vi "CfgManager.Text.INI Test Launcher.vi"() -> ()   [LabVIEW 2013]
uses:
  source/Manager.Text.INI/ConfigManager.Text.INI.lvclass
  <vilib>/LabVIEW Open Source Project/Data Manipulation/TypeDescriptor/TypeDescriptor_GetName.vi
  <vilib>/LabVIEW Open Source Project/Data Manipulation/TypeDescriptor/TypeDescriptor_GetPString.vi
  source/Manager/Decompose KVPs.vi
  source/Manager/Write.vi
  source/Manager/ConfigManager.lvclass
  <vilib>/LabVIEW Open Source Project/Data Manipulation/Variant/OpenVariant.lvlib
panel:
  out "Settings":cluster{"P":dbl, "I":dbl, "D":dbl}
  out "_staticdeps":T1
  out "any found?":bool
  out "_dyndependencies":T2(array[cluster])
  out "Keys":string[](array[string])
  out "modified configuration":variant
  out "error out":errorcluster
  out "initial configuration":variant
  out "filepath":path
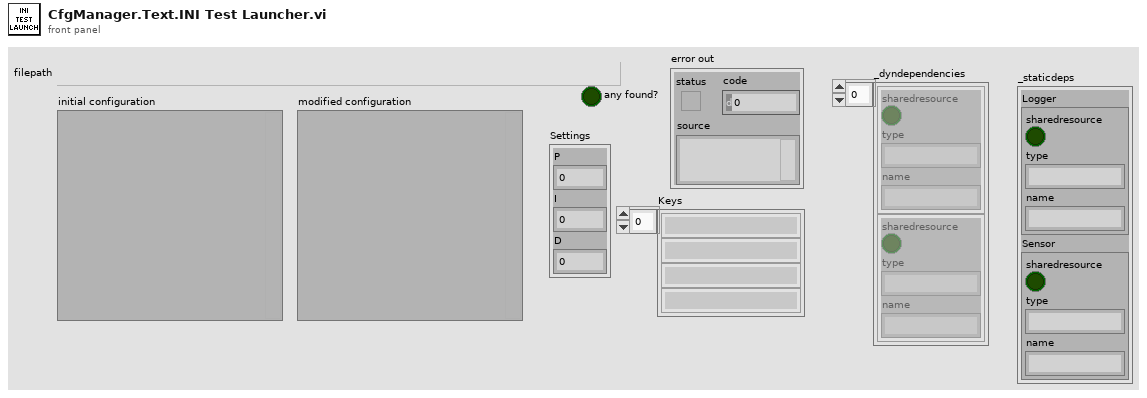
[diagram p1: front panel]
types:
  T1 = cluster{"Logger":cluster{"sharedresource":bool, "type":string, "name":string}, "Sensor":cluster{"sharedresource":bool, "type":string, "name":string}}
  T2 = cluster{"sharedresource":bool, "type":string, "name":string}[]
  T3 = cluster{"sharedresource":bool, "type":string, "name":string}
  T4 = cluster{"String":string, "Numeric":dbl, "Boolean":bool}
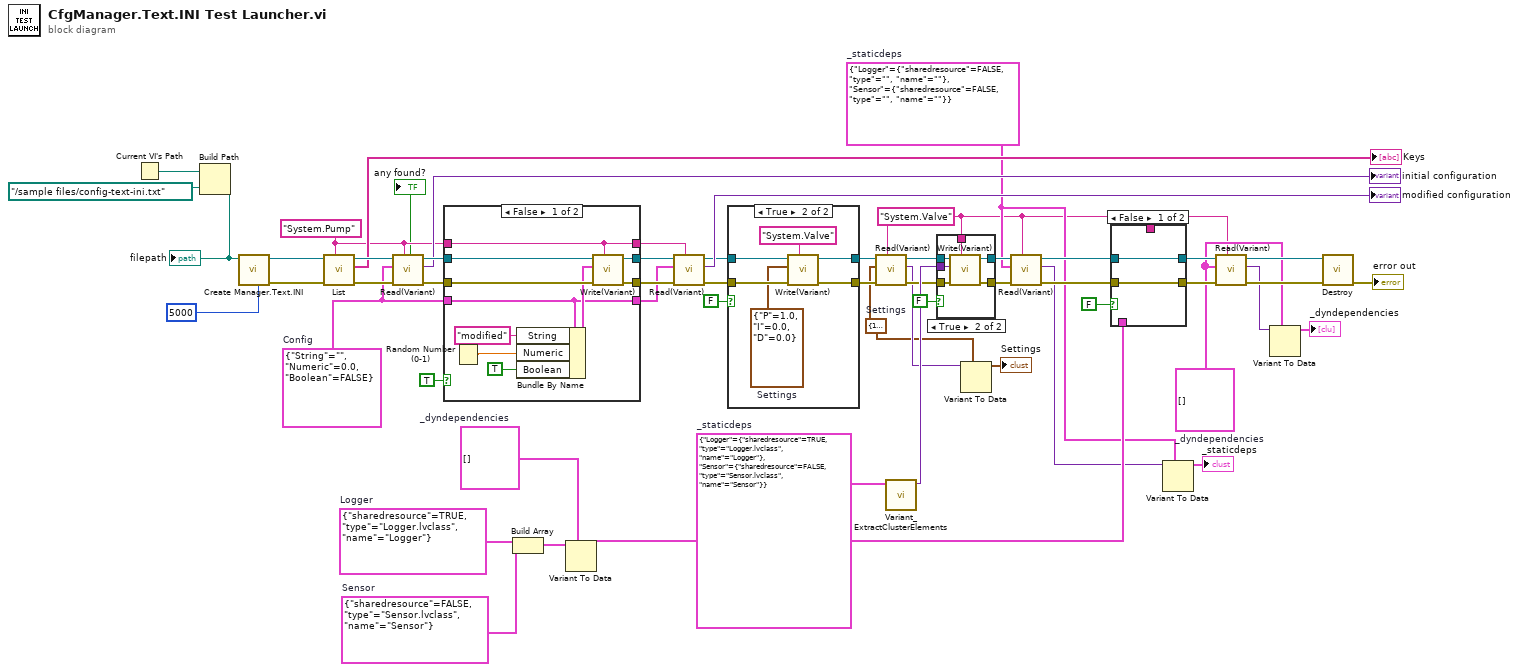
[diagram p0: block diagram]
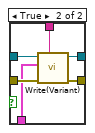
[diagram p3: hidden frame]
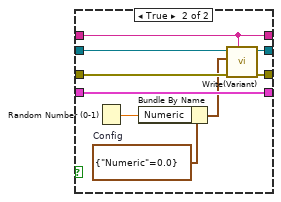
[diagram p4: hidden frame]
diagram:
  w2 = cluster{"P":dbl, "I":dbl, "D":dbl} {"P"=1.0, "I"=0.0, "D"=0.0}  # Settings
  w11 = T1 {"Logger"={"sharedresource"=FALSE, "type"="", "name"=""}, "Sensor"={"sharedresource"=FALSE, "type"="", "name"=""}}  # _staticdeps
  w21 = T2 []  # _dyndependencies
  w27 = T2 []  # _dyndependencies
  w29 = T3 {"sharedresource"=FALSE, "type"="Sensor.lvclass", "name"="Sensor"}  # Sensor
  w30 = T3 {"sharedresource"=TRUE, "type"="Logger.lvclass", "name"="Logger"}  # Logger
  w32 = T1 {"Logger"={"sharedresource"=TRUE, "type"="Logger.lvclass", "name"="Logger"}, "Sensor"={"sharedresource"=FALSE, "type"="Sensor.lvclass", "name"="Sensor"}}  # _staticdeps
  w6 = "System.Valve" ("Qualified Name")
  w43 = "System.Pump" ("Qualified Name")
  w40 = T4 {"String"="", "Numeric"=0.0, "Boolean"=FALSE}  # Config
  n1 = Current VI's Path() -> (path=w38:path)
  n2 = Build Path(base path=w38, name or relative path=path "../sample files/config-text-ini.txt" ("filepath 2")) -> (appended path=w36:path)
  "filepath" <- w36
  n3 = call "Create Manager.Text.INI.vi"("write delay (ms)"=5000, "filepath"=w36) -> ("error out"=w34:errorcluster, "ConfigManager.Text.INI out"=w35:refnum<class "ConfigManager.Text.INI.lvclass">)  [unwired: 7 in, 1 out]
  n4 = call "List.vi"("Qualified Name"=w43, "error in (no error)"=w34, "ConfigManager in"=w35) -> ("error out"=w50:errorcluster, "Keys"=→"Keys":string[], "ConfigManager out"=w49:refnum<class "ConfigManager.Text.INI.lvclass">)  [unwired: 6 in]
  n5 = call "Read(Variant).vi"("Qualified Name"=w43, "error in (no error)"=w50, "Type"=w40, "ConfigManager in"=w49) -> ("error out"=w54:errorcluster, "value"=→"initial configuration":variant, "ConfigManager out"=w55:refnum<class "ConfigManager.Text.INI.lvclass">, "any found?"=→"any found?":bool)  [unwired: 3 in, 1 out]
  n6 = case shown="False" TRUE {
    tunnel: w55 -> [w63 w75]
    tunnel: w54 -> [w62 w74]
    tunnel: [w65 w73] -> w53
    tunnel: [w64 w72] -> w52
    tunnel: w43 -> [w66 w71]
    tunnel: [w66 w71] -> w41
    tunnel: w40 -> [w57 w70]
    tunnel: [w57 w70] -> w39
    frame False {
      n7 = Random Number (0-1)() -> (number: 0 to 1=w59:dbl)
      n8 = Bundle By Name(cluster=w57, "String"="modified", "Numeric"=w59, "Boolean"=TRUE) -> (w58:T4)
      n9 = call "Write(Variant).vi"("Qualified Name"=w66, "error in (no error)"=w62, "value"=w58, "ConfigManager in"=w63) -> ("error out"=w64:errorcluster, "ConfigManager out"=w65:refnum<class "ConfigManager.Text.INI.lvclass">)  [unwired: 5 in, 1 out]
    }
    frame True {
      w69 = cluster{"Numeric":dbl} {"Numeric"=0.0}  # Config
      n10 = Random Number (0-1)() -> (number: 0 to 1=w68:dbl)
      n11 = Bundle By Name(cluster=w69, "Numeric"=w68) -> (w67:cluster{"Numeric":dbl})
      n12 = call "Write(Variant).vi"("Qualified Name"=w71, "error in (no error)"=w74, "value"=w67, "ConfigManager in"=w75) -> ("error out"=w72:errorcluster, "ConfigManager out"=w73:refnum<class "ConfigManager.Text.INI.lvclass">)  [unwired: 5 in, 1 out]
    }
  }
  n13 = Build Array(w30, w29) -> (w28:T2)
  n14 = Variant To Data(type=w27, Variant=w28) -> (data=w26:T2)  [unwired: 1 in, 1 out]
  n15 = call "Read(Variant).vi"("Qualified Name"=w41, "error in (no error)"=w52, "Type"=w39, "ConfigManager in"=w53) -> ("error out"=w45:errorcluster, "value"=→"modified configuration":variant, "ConfigManager out"=w46:refnum<class "ConfigManager.Text.INI.lvclass">)  [unwired: 3 in, 2 out]
  n16 = case shown="True" FALSE {
    tunnel: w46 -> [w77 w83]
    tunnel: [w77 w82] -> w7
    tunnel: w45 -> [w76 w81]
    tunnel: [w76 w80] -> w4
    frame False {
    }
    frame True {
      w78 = cluster{"P":dbl, "I":dbl, "D":dbl} {"P"=1.0, "I"=0.0, "D"=0.0}  # Settings
      n17 = call "Write(Variant).vi"("Qualified Name"="System.Valve", "error in (no error)"=w81, "value"=w78, "ConfigManager in"=w83) -> ("error out"=w80:errorcluster, "ConfigManager out"=w82:refnum<class "ConfigManager.Text.INI.lvclass">)  [unwired: 5 in, 1 out]
    }
  }
  n18 = call "Read(Variant).vi"("Qualified Name"=w6, "error in (no error)"=w4, "Type"=w2, "ConfigManager in"=w7) -> ("error out"=w5:errorcluster, "value"=w3:variant, "ConfigManager out"=w8:refnum<class "ConfigManager.Text.INI.lvclass">)  [unwired: 3 in, 2 out]
  n19 = call <vilib>:"Variant_ExtractClusterElements.vi"("Cluster"=w32) -> ("Cluster dup"=w31:variant)  [unwired: 8 in, 2 out]
  n20 = case shown="True" FALSE {
    tunnel: w8 -> [w85 w91]
    tunnel: w5 -> [w84 w90]
    tunnel: w31 -> [_ w89]
    tunnel: [w85 w88] -> w16
    tunnel: [w84 w87] -> w14
    tunnel: w6 -> [_ w86]
    frame False {
    }
    frame True {
      n21 = call "Write(Variant).vi"("Qualified Name"=w86, "error in (no error)"=w90, "value"=w89, "ConfigManager in"=w91) -> ("error out"=w87:errorcluster, "ConfigManager out"=w88:refnum<class "ConfigManager.Text.INI.lvclass">)  [unwired: 5 in, 1 out]
    }
  }
  n22 = Variant To Data(type=w2, Variant=w3) -> (data=→"Settings":cluster{"P":dbl, "I":dbl, "D":dbl})  [unwired: 1 in, 1 out]
  n23 = call "Read(Variant).vi"("Qualified Name"=w6, "error in (no error)"=w14, "Type"=w11, "ConfigManager in"=w16) -> ("error out"=w13:errorcluster, "value"=w12:variant, "ConfigManager out"=w15:refnum<class "ConfigManager.Text.INI.lvclass">)  [unwired: 3 in, 2 out]
  n24 = case shown="False" FALSE {
    tunnel: w15 -> [w93 w99]
    tunnel: w13 -> [w92 w98]
    tunnel: w26 -> [_ w97]
    tunnel: [w93 w96] -> w25
    tunnel: [w92 w95] -> w23
    tunnel: w6 -> [_ w94]
    frame False {
    }
    frame True {
      n25 = call "Write(Variant).vi"("Qualified Name"=w94, "error in (no error)"=w98, "value"=w97, "ConfigManager in"=w99) -> ("error out"=w95:errorcluster, "ConfigManager out"=w96:refnum<class "ConfigManager.Text.INI.lvclass">)  [unwired: 5 in, 1 out]
    }
  }
  n26 = Variant To Data(type=w11, Variant=w12) -> (data=→"_staticdeps":T1)  [unwired: 1 in, 1 out]
  n27 = call "Read(Variant).vi"("Qualified Name"=w6, "error in (no error)"=w23, "Type"=w21, "ConfigManager in"=w25) -> ("error out"=w22:errorcluster, "value"=w20:variant, "ConfigManager out"=w24:refnum<class "ConfigManager.Text.INI.lvclass">)  [unwired: 3 in, 2 out]
  n28 = Variant To Data(type=w21, Variant=w20) -> (data=→"_dyndependencies":T2)  [unwired: 1 in, 1 out]
  n29 = call-dynamic "Destroy.vi"("error in (no error)"=w22, "ConfigManager.Text in"=w24) -> ("error out"=→"error out":errorcluster)  [unwired: 8 in, 1 out]
